vi "abre_HELP.vi"(1 "nome":string) -> (0 "Erro":bool)   [LabVIEW 2019]
doc: "Este vi abre arquivos pelo Acrobat (.pdf).\nNome PDF - nome do arquivo que deseja abrir. Ele deve estar na subpasta data do mesmo diretório que este vi.\nOk - se false é pq ocorreu algum erro ao procurar o arquivo. Para saber qual erro ocorreu, veja em error out. Caso contrário, o arquivo é aberto."
panel:
  out "error out":errorcluster
  in  "error in (no error)":errorcluster
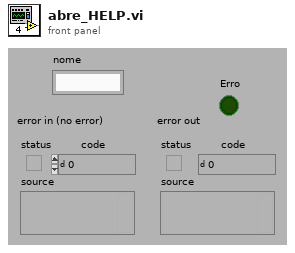
[diagram p1: front panel]
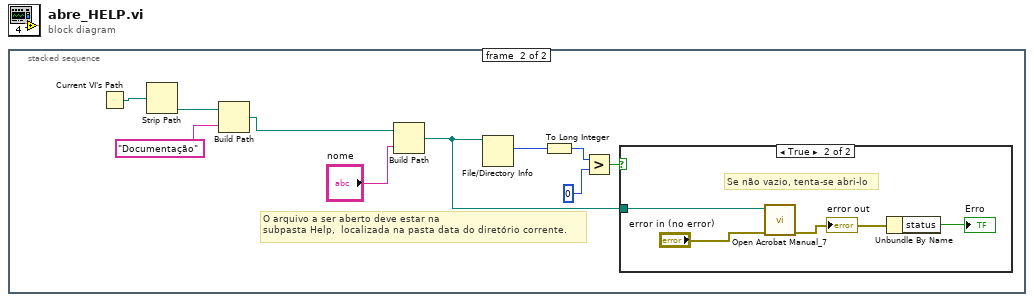
[diagram p0: block diagram]
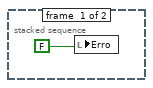
[diagram p2: hidden frame]
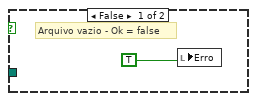
[diagram p3: hidden frame]
diagram:
  n1 = stacked-sequence {
    frame #0 {
      n2 = local write "Erro"(FALSE) -> ()
    }
    frame #1 {
      # "O arquivo a ser aberto deve estar na \nsubpasta Help,  localizada na pasta data do diretório corrente."
      n3 = Current VI's Path() -> (path=w6:path)
      n4 = Strip Path(path=w6) -> (stripped path=w5:path)  [unwired: 1 out]
      n5 = Build Path(base path=w5, name or relative path="Documentação") -> (appended path=w3:path)
      n6 = Build Path(base path=w3, name or relative path="nome") -> (appended path=w2:path)
      n7 = File/Directory Info(path=w2) -> (size=w7:i64)  [unwired: 1 in, 6 out]
      n8 = To Long Integer(number=w7) -> (32bit integer=w9:i32)
      n9 = Greater?(x=w9, y=0) -> (0:w11:bool)
      n10 = case shown="True" w11 {
        tunnel: w2 -> [_ w16]
        frame False {
          # "Arquivo vazio - Ok = false"
          n11 = local write "Erro"(TRUE) -> ()
        }
        frame True {
          # "Se não vazio, tenta-se abri-lo"
          n12 = call "Open Acrobat Manual_7.vi"("error in (no error)"="error in (no error)", "acrobat document"=w16) -> ("error out"=w14:errorcluster)  [unwired: 5 in]
          "error out" <- w14
          n13 = Unbundle By Name(w14) -> ("status"=→"Erro":bool)
        }
      }
    }
  }
